vi "PXF4_get_PV_MV.vi"(7 "delay":dbl=0.01 caption="Delay Time (s)", 8 "error in":errorcluster, 11 "Modbus Master in":refnum<class "Modbus Master.lvclass">) -> (0 "error out":errorcluster, 1 "SV":dbl format="%.1f", 2 "PV":dbl format="%.1f", 3 "Modbus Master out":refnum<class "Modbus Master.lvclass">, 4 "Output":bool)   [LabVIEW 2019]
uses:
  <vilib>/NI/Modbus Library/API/Master/Modbus Master.lvclass
panel:
  out "MV1":u16
  out "SV_raw":u16
  out "PV_raw":u16
  out "register values":u16[](array[numeric])
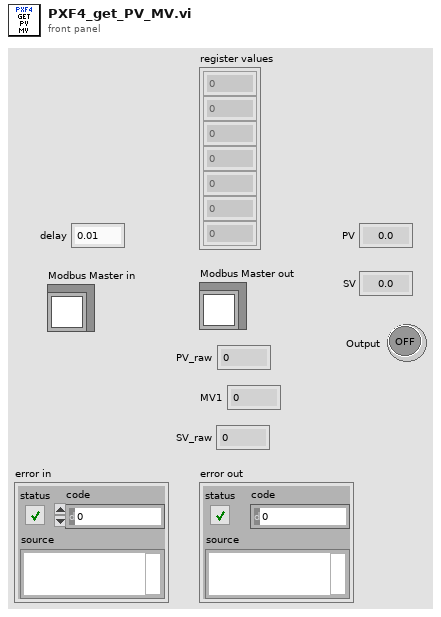
[diagram p1: front panel]
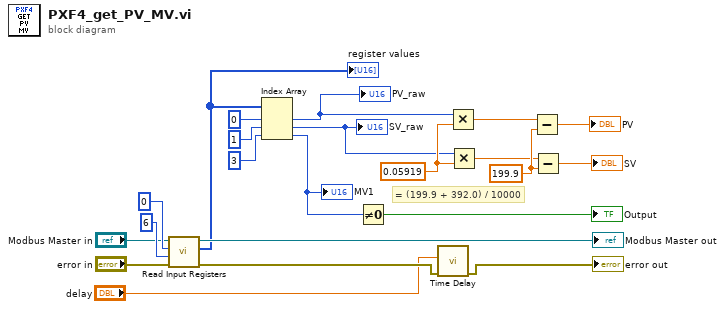
[diagram p0: block diagram]
diagram:
  w8 = 199.9 ("y")
  w11 = 0.05919 ("y")
  # "= (199.9 + 392.0) / 10000"
  n1 = call-dynamic "Read Input Registers.vi"("error in"="error in", "number of inputs"=u16 6, "starting address"=u16 0, "Modbus master in"="Modbus Master in") -> ("error out"=w3:errorcluster, "register values"=w18:u16[], "Modbus master out"=→"Modbus Master out":refnum<class "Modbus Master.lvclass">)  [unwired: 5 in]
  "register values" <- w18
  n2 = Index Array(array=w18, index #1=0 ("index"), index #2=1 ("index"), index #3=3 ("index")) -> (element #1=w9:u16, element #2=w10:u16, element #3=w13:u16)
  "PV_raw" <- w9
  "SV_raw" <- w10
  "MV1" <- w13
  n3 = Not Equal To 0?(x=w13) -> (x != 0?=→"Output":bool)
  n4 = call "Time Delay"("error in (no error)"=w3, "Delay Time (s)"="delay") -> ("error out"=→"error out":errorcluster)  [unwired: 9 in]
  n5 = Multiply(x=w9, y=w11) -> (x*y=w7:dbl)
  n6 = Multiply(x=w10, y=w11) -> (x*y=w6:dbl)
  n7 = Subtract(x=w7, y=w8) -> (x-y=→"PV":dbl)
  n8 = Subtract(x=w6, y=w8) -> (x-y=→"SV":dbl)
